vi "CommandFIFO6.vi"   [LabVIEW 2016]
uses:
  <vilib>/rvi/Emulation/niFpgaGetClockAttributes.vi
  <vilib>/rvi/Emulation/niFpgaSctlEmulationGetInTimedLoop.vi
  <vilib>/rvi/Emulation/niFpgaEmulationReportErrorSimple.vi
  <vilib>/rvi/interface/RandomDataEmulation/niFpgaRandomDataHandleErrors.vi
  <vilib>/rvi/DataTransferAndStorage/Container/Common/niFpgaContainerExecOnDevCompGetState.vi
  <vilib>/rvi/Emulation/niFpgaEmulationIsFPGAContextNoSignature.vi
  <vilib>/rvi/errors/niFpgaSetErrorForExecOnDevCompSimple.vi
  <vilib>/rvi/eio/common/nirviEmuReportErrorAndStop.vi
  <vilib>/rvi/DataTransferAndStorage/Container/Common/niFpgaContainerGetUniqueNameForEmu.vi
  <vilib>/rvi/FIFO/Fifo_Resource/nirvififoEmulationSetSize.vi
  <vilib>/rvi/FIFO/Fifo_Resource/nirviFifoEmulationQueueMgr.vi
  <instcachedir>/0/nirviFifoEmulationQueueMgr_E5CAEC123FF24DC58D834DCA3CDAA9B5.lvgen/nirviFifoEmulationQueueMgr_E5CAEC123FF24DC58D834DCA3CDAA9B5_002.vi
  <vilib>/rvi/FIFO/Fifo_Resource/nirvififoEmulationDetermineInputValidOut.vi
  <vilib>/rvi/FIFO/Fifo_Resource/nirvififoEmulationCreateLock.vi
  <vilib>/rvi/Emulation/niFpgaProcessEmulError.vi
  <vilib>/rvi/FIFO/Fifo_Resource/nirvififoEmulationObtainLock.vi
  <vilib>/rvi/FIFO/Fifo_Resource/nirvififoEmulationReleaseLock.vi
  <vilib>/rvi/occurrence/nirviWaitOnOccurrenceBase.vi
  <vilib>/rvi/errors/nirviReportUnexpectedCaseInternalError.vi
  <vilib>/rvi/errors/nirviReportUnexpectedCaseInternalError (U32).vi
  <vilib>/Utility/error.llb/Clear Errors.vi
  <vilib>/rvi/eio/common/nirviEmuTemplateMethod_errors.vi
  <instcachedir>/0/nirviFifoEmulationQueueMgr_E5CAEC123FF24DC58D834DCA3CDAA9B5.lvgen/nirviFifoEmulationQueueMgr_E5CAEC123FF24DC58D834DCA3CDAA9B5_007.vi
  <vilib>/rvi/Emulation/niFpgaCriticalErrorInLSC.vi
  <vilib>/rvi/DataTransferAndStorage/Container/XNode/niFpgaContainer.xnode
  <vilib>/rvi/interface/RandomDataEmulation/nirviRandomDataFpgaReadWriteTemplate.vi
  <vilib>/rvi/FIFO/Fifo_Resource/niFpgaFifoEmulationRefIn.vi
  <vilib>/eio/EIONode/EIONode.xnode
  <vilib>/rvi/FIFO/Fifo_Resource/nirvififoEmulationWrite.vi
types:
  T1 = typedef "Addresses.ctl" = enum8{"NA", "Accelerometer1X", "Accelerometer1Y", "Accelerometer1Z", "Accelerometer2X", "Accelerometer2Y", "Accelerometer2Z", "Accelerometer3X", "Accelerometer3Y", "Accelerometer3Z", "Accelerometer4X", "Accelerometer4Y", "Accelerometer4Z", "Accelerometer5X", "Accelerometer5Y", "Accelerometer5Z", "Accelerometer6X", "Accelerometer6Y", "Accelerometer6Z", "Sync1", "Sync2", "Sync3", "Sync4", "Accelerometer1", "Accelerometer2", "Accelerometer3", "Accelerometer4", "Accelerometer5", "Accelerometer6", "Accelerometers", "Timestamp", "SamplePeriod"}
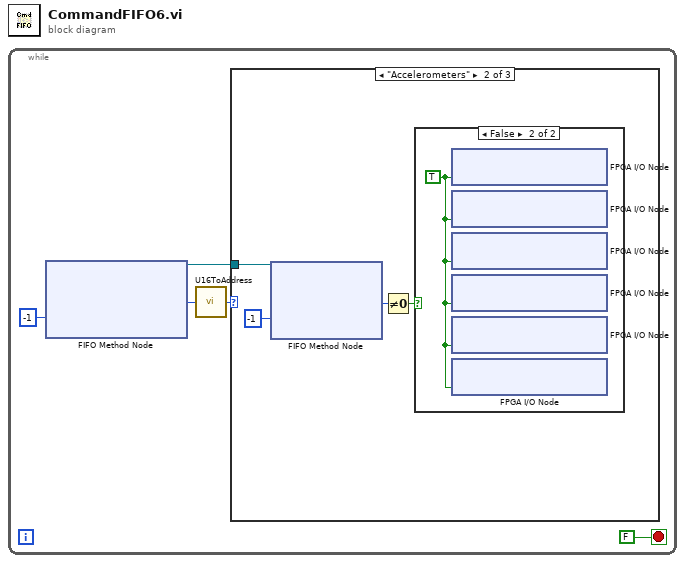
[diagram p0: block diagram]
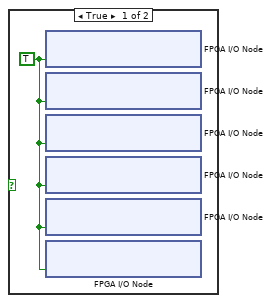
[diagram p3: hidden frame]
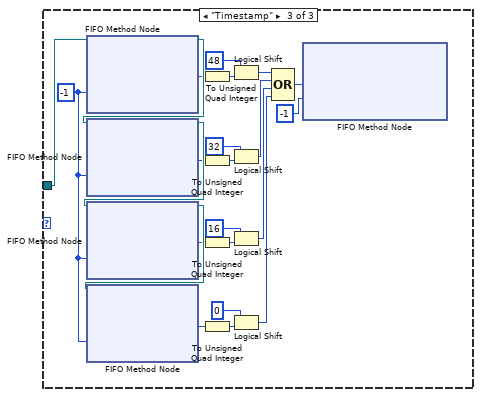
[diagram p4: hidden frame]
diagram:
  n1 = while {
    stop <- FALSE stop-if-true
    n2 = xnode ("FIFO Method Node")("Timeout"=-1) -> ("Element"=w3:u16, "FIFO Out"=w1:refnum<k21>)  [unwired: 1 in, 1 out]
    n3 = call "U16ToAddress.vi"("Input"=w3) -> ("Addresses"=w2:T1)
    n4 = case shown="\"Accelerometers\"" w2 {
      tunnel: w1 -> [_ w9 w31]
      frame "NA", Default {
      }
      frame "Accelerometers" {
        n5 = xnode ("FIFO Method Node")("Timeout"=-1, "FIFO In"=w9) -> ("Element"=w7:u16)  [unwired: 2 out]
        n6 = Not Equal To 0?(x=w7) -> (x != 0?=w6:bool)
        n7 = case shown="False" w6 {
          frame True {
            w10 = TRUE ("Accelerometer5/Start")
            n8 = xnode "FPGA I/O Node"("Accelerometer1/Start"=w10) -> ()  [unwired: 1 in, 1 out]
            n9 = xnode "FPGA I/O Node"("Accelerometer2/Start"=w10) -> ()  [unwired: 1 in, 1 out]
            n10 = xnode "FPGA I/O Node"("Accelerometer3/Start"=w10) -> ()  [unwired: 1 in, 1 out]
            n11 = xnode "FPGA I/O Node"("Accelerometer4/Start"=w10) -> ()  [unwired: 1 in, 1 out]
            n12 = xnode "FPGA I/O Node"("Accelerometer5/Start"=w10) -> ()  [unwired: 1 in, 1 out]
            n13 = xnode "FPGA I/O Node"("Accelerometer6/Start"=w10) -> ()  [unwired: 1 in, 1 out]
          }
          frame False {
            w11 = TRUE ("Accelerometer5/Start")
            n14 = xnode "FPGA I/O Node"("Accelerometer1/Stop"=w11) -> ()  [unwired: 1 in, 1 out]
            n15 = xnode "FPGA I/O Node"("Accelerometer2/Stop"=w11) -> ()  [unwired: 1 in, 1 out]
            n16 = xnode "FPGA I/O Node"("Accelerometer3/Stop"=w11) -> ()  [unwired: 1 in, 1 out]
            n17 = xnode "FPGA I/O Node"("Accelerometer4/Stop"=w11) -> ()  [unwired: 1 in, 1 out]
            n18 = xnode "FPGA I/O Node"("Accelerometer5/Stop"=w11) -> ()  [unwired: 1 in, 1 out]
            n19 = xnode "FPGA I/O Node"("Accelerometer6/Stop"=w11) -> ()  [unwired: 1 in, 1 out]
          }
        }
      }
      frame "Timestamp" {
        w30 = -1 ("Timeout")
        n20 = xnode ("FIFO Method Node")("Timeout"=w30, "FIFO In"=w31) -> ("Element"=w29:u16, "FIFO Out"=w34:refnum<k21>)  [unwired: 1 out]
        n21 = xnode ("FIFO Method Node")("Timeout"=w30, "FIFO In"=w34) -> ("Element"=w28:u16, "FIFO Out"=w33:refnum<k21>)  [unwired: 1 out]
        n22 = xnode ("FIFO Method Node")("Timeout"=w30, "FIFO In"=w33) -> ("Element"=w27:u16, "FIFO Out"=w32:refnum<k21>)  [unwired: 1 out]
        n23 = xnode ("FIFO Method Node")("Timeout"=w30, "FIFO In"=w32) -> ("Element"=w26:u16)  [unwired: 2 out]
        n24 = To Unsigned Quad Integer(1:w29) -> (0:w25:u64)
        n25 = To Unsigned Quad Integer(1:w28) -> (0:w24:u64)
        n26 = To Unsigned Quad Integer(1:w27) -> (0:w23:u64)
        n27 = To Unsigned Quad Integer(1:w26) -> (0:w22:u64)
        n28 = Logical Shift(y=i16 48, x=w25) -> (x << y=w17:u64)
        n29 = Logical Shift(y=i16 32, x=w24) -> (x << y=w16:u64)
        n30 = Logical Shift(y=i16 16, x=w23) -> (x << y=w15:u64)
        n31 = Logical Shift(y=i16 0, x=w22) -> (x << y=w14:u64)
        n32 = Compound Arithmetic op=OR(w17, w16, w15, w14) -> (w13:u64)
        n33 = xnode ("FIFO Method Node")("Element"=w13, "Timeout"=-1) -> ()  [unwired: 1 in, 2 out]
      }
    }
  }
